vi "hioki.vi"(6 "TimeOut":u32=1000, 7 "PWA(V)":dbl, 8 "error in (no error)":errorcluster, 9 "Clu_SEQ":T1, 10 "EnumFunction":T2(ring), 11 "VISA resource name out":refnum<visa-resource-name>="COM2") -> (0 "error out":errorcluster, 2 "read buffer":string, 3 "Visa_HiokiMeterOut":refnum<visa-resource-name>)   [LabVIEW 2016]
uses:
  <vilib>/Instr/_visa.llb/VISA Open Access Mode.ctl
panel:
  out "x >= y?":bool
  out "sum":u32
  out "x-y":u32
  out "MeassuredValue":dbl format="%#_6e"
  out "ComparisonResult":i32
  out "Status":i32
  out "ch":i32
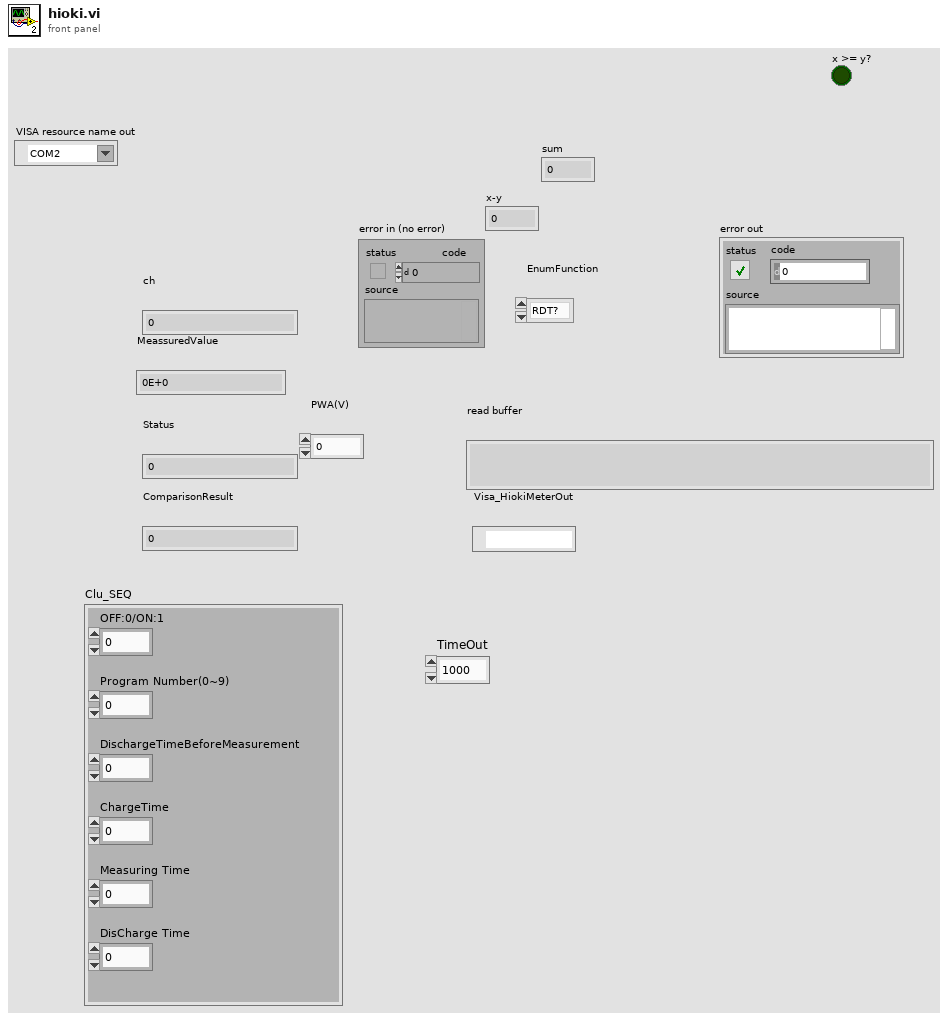
[diagram p1: front panel]
types:
  T1 = cluster{"OFF:0/ON:1":i32, "Program Number(0~9)":i32, "DischargeTimeBeforeMeasurement":dbl, "ChargeTime":dbl, "Measuring Time":dbl, "DisCharge Time":dbl}
  T2 = enum16{"RDT?", "IDN?", "SRT", "CBF", "SEQ?", "RMT", "SEQ", "PWS", "STP", "PWS?", "PWA", "CHS", ""}
  T3 = typedef "VISA Open Access Mode.ctl" = u32
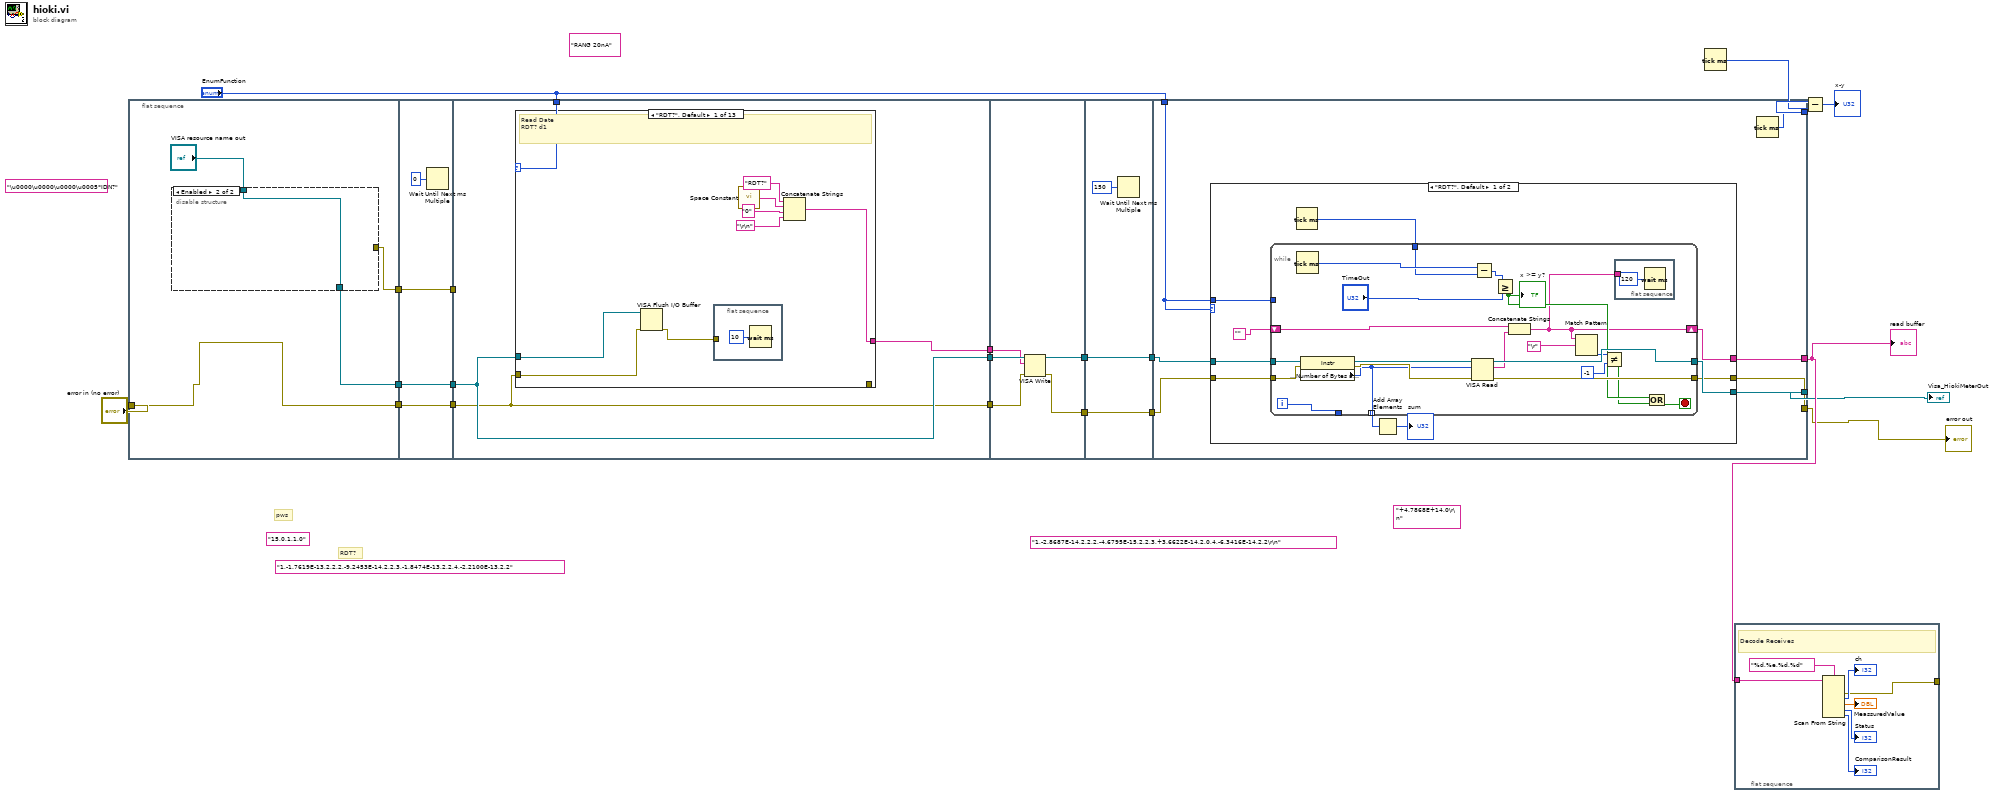
[diagram p0: block diagram]
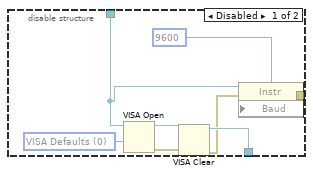
[diagram p2: hidden frame]
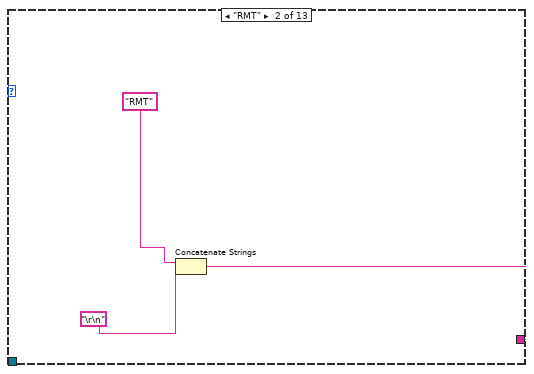
[diagram p3: hidden frame]
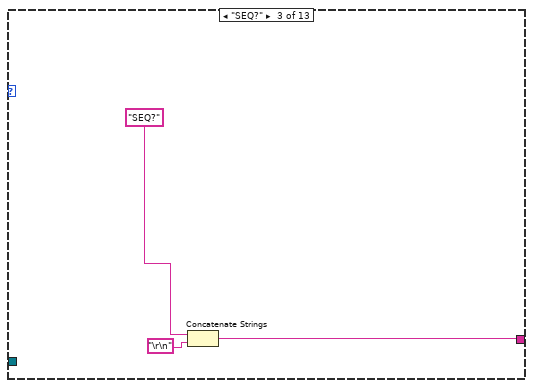
[diagram p4: hidden frame]
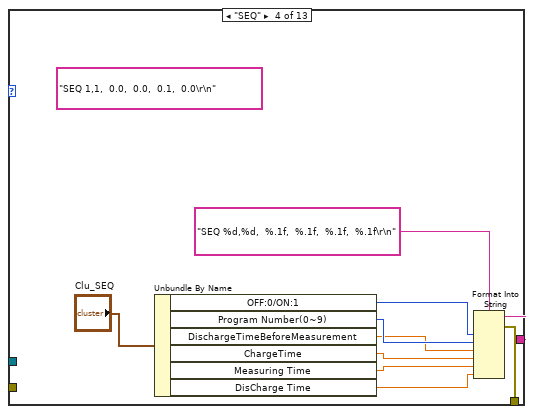
[diagram p5: hidden frame]
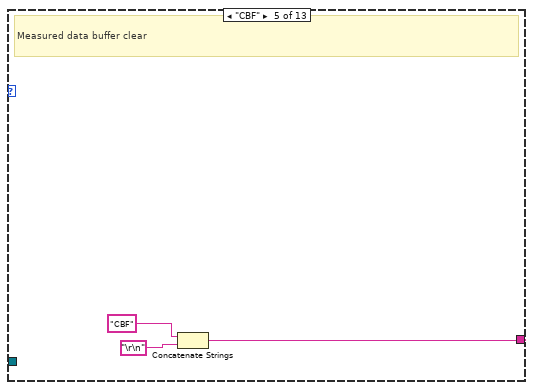
[diagram p6: hidden frame]
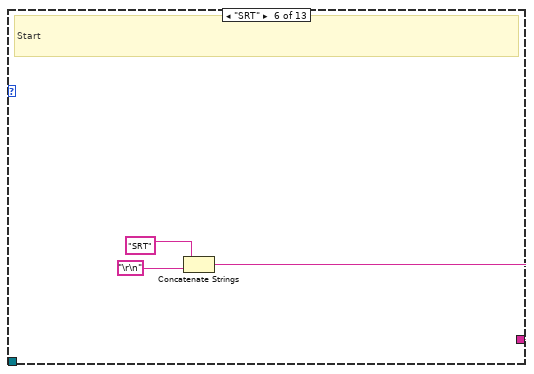
[diagram p7: hidden frame]
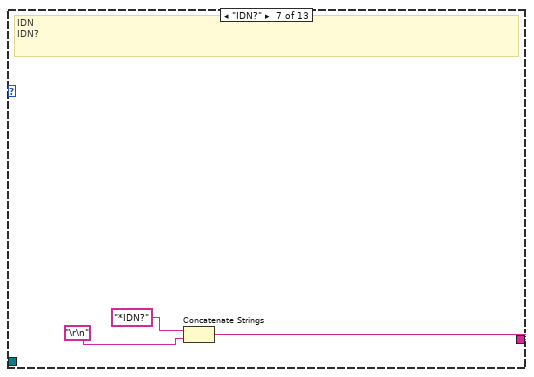
[diagram p8: hidden frame]
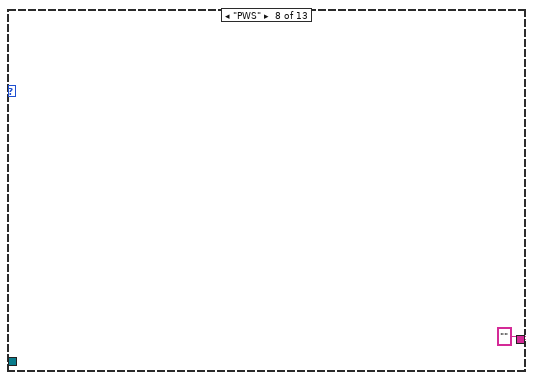
[diagram p9: hidden frame]
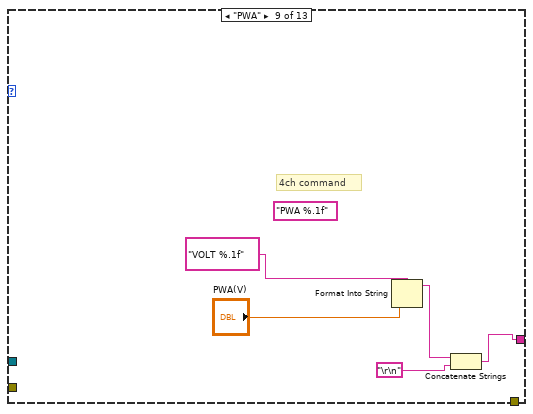
[diagram p10: hidden frame]
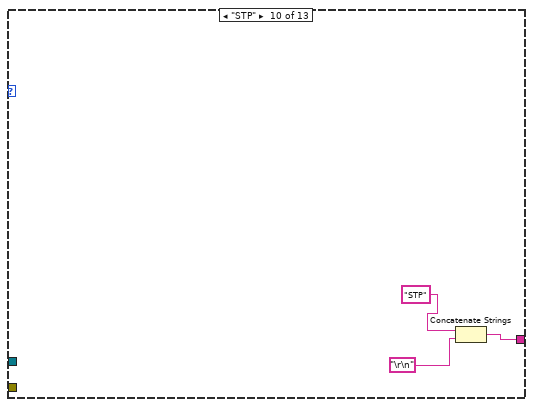
[diagram p11: hidden frame]
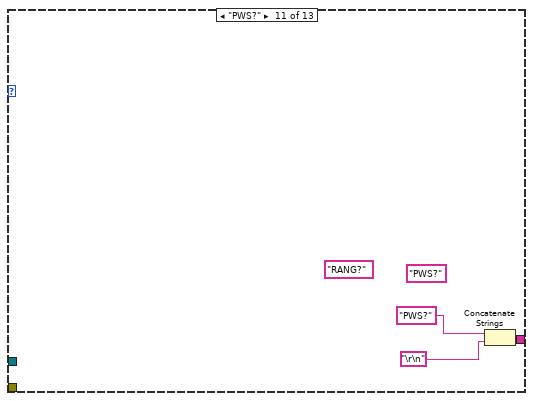
[diagram p12: hidden frame]
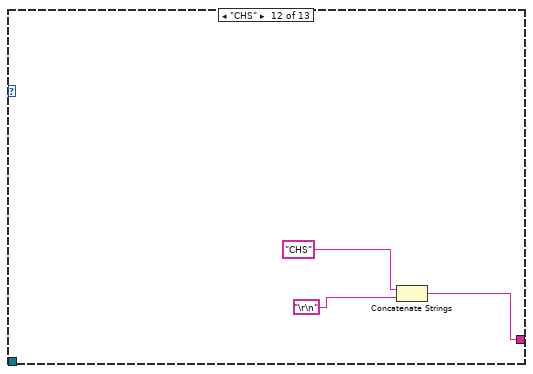
[diagram p13: hidden frame]
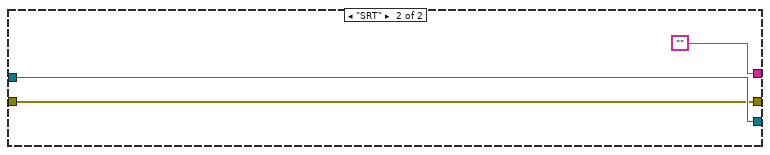
[diagram p15: hidden frame]
diagram:
  (unwired) "RANG 20nA"
  (unwired) "+4.7868E+14,0\r\n" ("read buffer 2")
  (unwired) "1,-2.8687E-14,2,2,2,-4.6795E-15,2,2,3,+3.6622E-14,2,0,4,-6.3416E-14,2,2\r\n" ("read buffer")
  (unwired) "1,-1.7619E-13,2,2,2,-9.2453E-14,2,2,3,-1.8474E-13,2,2,4,-2.2100E-13,2,2"
  (unwired) "15,0,1,1,0"
  (unwired) "\u0000\u0000\u0000\u0005*IDN?" ("Display")
  # "RDT?"
  # "pws"
  n1 = flat-sequence {
    tunnel: [w25] -> w8
    tunnel: [w24] -> w6
    tunnel: "error in (no error)" -> [w25]
    tunnel: [w22] -> w4
    tunnel: w8 -> [w38]
    tunnel: [w38] -> w7
    tunnel: w6 -> [w37]
    tunnel: [w37] -> w5
    tunnel: w4 -> [w36]
    tunnel: [w36] -> w3
    tunnel: w7 -> [w40]
    tunnel: w5 -> [w41]
    tunnel: "EnumFunction" -> [w42]
    tunnel: [w41] -> w18
    tunnel: [w40] -> w17
    tunnel: [w39] -> w14
    tunnel: w3 -> [_]
    tunnel: [w95] -> w19
    tunnel: w18 -> [w96]
    tunnel: w17 -> [w94]
    tunnel: [w93] -> w16
    tunnel: w14 -> [w92]
    tunnel: w19 -> [w99]
    tunnel: [w99] -> w21
    tunnel: w16 -> [w97]
    tunnel: [w97] -> w15
    tunnel: w21 -> [w106]
    tunnel: [w105] -> w2
    tunnel: [w104] -> w1
    tunnel: w15 -> [w103]
    tunnel: [w102] -> w9
    tunnel: "EnumFunction" -> [w101]
    tunnel: [w100] -> w12
    frame #0 {
      n2 = disable-structure shown="Enabled" {
        disable-tunnel: [w33 w34] -> w24
        disable-tunnel: "VISA resource name out" -> [w32 w34]
        disable-tunnel: [w31 _] -> w22
        frame Disabled {
          w28 = T3 0 items=["VISA Defaults"=0, "Exclusive Lock"=1, "Load Configured Settings"=4] ("Access Mode")
          n3 = VISA Open(access mode=w28, VISA resource name=w32) -> (VISA resource name=w30:refnum<visa-resource-name>, error out=w29:errorcluster)  [unwired: 3 in]
          n4 = VISA Clear(VISA resource name=w30, error in (no error)=w29) -> (VISA resource name out=w33:refnum<visa-resource-name>, error out=w26:errorcluster)
          n5 = property class="Instr"(reference=w32, error in=w26, "Baud"=u32 9600 ("Serial Settings:Baud Rate")) -> (error out=w31:errorcluster)  [unwired: 1 out]
        }
        frame Enabled {
        }
      }
    }
    frame #1 {
      n6 = Wait Until Next ms Multiple(millisecond multiple=u32 0) -> ()  [unwired: 1 out]
    }
    frame #2 {
      n7 = case shown="\"RDT?\", Default" w42 {
        tunnel: [w48 w53 w55 w66 w69 w72 w76 "" w79 w85 w86 w89 _] -> w39
        tunnel: [_ _ _ w65 _ _ _ _ _ _ _ _ _] -> _
        tunnel: w41 -> [w45 _ _ _ _ _ _ _ _ _ _ _ _]
        tunnel: w40 -> [w44 _ _ _ _ _ _ _ _ _ _ _ _]
        frame "RDT?", Default {
          # "Read Date\nRDT? d1"
          n8 = VISA Flush I/O Buffer(VISA resource name=w45, error in (no error)=w44) -> (error out=w43:errorcluster)  [unwired: 1 in, 1 out]
          n9 = flat-sequence {
            tunnel: w43 -> [_]
            frame #0 {
              n10 = Wait (ms)(milliseconds to wait=u32 10) -> ()  [unwired: 1 out]
            }
          }
          n11 = call <vilib>:"Space Constant.vi"() -> ("String"=w49:string)
          n12 = Concatenate Strings("RDT?", w49, "0" ("string"), "\r\n") -> (w48:string)
        }
        frame "RMT" {
          n13 = Concatenate Strings("RMT", "\r\n") -> (w53:string)
        }
        frame "SEQ?" {
          n14 = Concatenate Strings("SEQ?", "\r\n") -> (w55:string)
        }
        frame "SEQ" {
          (unwired) "SEQ 1,1,  0.0,  0.0,  0.1,  0.0\r\n" ("read buffer")
          n15 = Unbundle By Name("Clu_SEQ") -> ("OFF:0/ON:1"=w63:i32, "Program Number(0~9)"=w62:i32, "DischargeTimeBeforeMeasurement"=w61:dbl, "ChargeTime"=w60:dbl, "Measuring Time"=w59:dbl, "DisCharge Time"=w58:dbl)
          n16 = Format Into String(format string="SEQ %d,%d,  %.1f,  %.1f,  %.1f,  %.1f\r\n" ("read buffer"), w63, w62, w61, w60, w59, w58) -> (resulting string=w66:string, error out=w65:errorcluster)  [unwired: 2 in]
        }
        frame "CBF" {
          # "Measured data buffer clear"
          n17 = Concatenate Strings("CBF", "\r\n") -> (w69:string)
        }
        frame "SRT" {
          # "Start"
          n18 = Concatenate Strings("SRT", "\r\n") -> (w72:string)
        }
        frame "IDN?" {
          # "IDN \nIDN?"
          n19 = Concatenate Strings("*IDN?", "\r\n") -> (w76:string)
        }
        frame "PWS" {
        }
        frame "PWA" {
          (unwired) "PWA %.1f"
          # "4ch command"
          n20 = Format Into String(format string="VOLT %.1f", "PWA(V)") -> (resulting string=w81:string)  [unwired: 2 in, 1 out]
          n21 = Concatenate Strings(w81, "\r\n") -> (w79:string)
        }
        frame "STP" {
          n22 = Concatenate Strings("STP", "\r\n") -> (w85:string)
        }
        frame "PWS?" {
          (unwired) "RANG?"
          (unwired) "PWS?"
          n23 = Concatenate Strings("PWS?", "\r\n") -> (w86:string)
        }
        frame "CHS" {
          n24 = Concatenate Strings("CHS", "\r\n") -> (w89:string)
        }
        frame "" {
        }
      }
    }
    frame #3 {
      n25 = VISA Write(VISA resource name=w96, write buffer=w92, error in (no error)=w94) -> (VISA resource name out=w93:refnum<visa-resource-name>, error out=w95:errorcluster)  [unwired: 1 out]
    }
    frame #4 {
      n26 = Wait Until Next ms Multiple(millisecond multiple=u32 150) -> ()  [unwired: 1 out]
    }
    frame #5 {
      n27 = case shown="\"RDT?\", Default" w101 {
        tunnel: w106 -> [w116 w140]
        tunnel: [w115 w141] -> w105
        tunnel: [w114 w140] -> w104
        tunnel: w103 -> [w113 w141]
        tunnel: [w110 ""] -> w102
        tunnel: w101 -> [w109 _]
        frame "RDT?", Default {
          n28 = Tick Count (ms)() -> (millisecond timer value=w112:u32)
          n29 = while {
            tunnel: w112 -> [w130]
            tunnel: w116 -> [w137]
            tunnel: [w133] -> w114
            shift-right: [w118] -> w110
            shift-left: "" -> [w126]
            tunnel: w109 -> [_]
            tunnel: w113 -> [w132]
            tunnel: [w134] -> w115
            tunnel: [w119] -> _
            tunnel: [w117] -> w108 mode=indexing
            i -> [w119]
            stop <- w121 stop-if-true
            n30 = Tick Count (ms)() -> (millisecond timer value=w131:u32)
            n31 = property class="Instr"(reference=w132, error in=w137) -> (reference out=w136:refnum<visa-resource-name>, error out=w135:errorcluster, "Serial Settings:Number of Bytes at Serial Port"=w117:u32)
            n32 = VISA Read(VISA resource name=w136, byte count=w117, error in (no error)=w135) -> (VISA resource name out=w134:refnum<visa-resource-name>, read buffer=w127:string, error out=w133:errorcluster)  [unwired: 1 out]
            n33 = Subtract(x=w131, y=w130) -> (x-y=w129:u32)
            n34 = Greater Or Equal?(x=w129, y="TimeOut") -> (x >= y?=w125:bool)
            "x >= y?" <- w125
            n35 = Concatenate Strings(w126, w127) -> (w118:string)
            n36 = Match Pattern(string=w118, regular expression="\r") -> (offset past match=w124:i32)  [unwired: 1 in, 3 out]
            n37 = Not Equal?(x=w124, y=-1) -> (x != y?=w122:bool)
            n38 = flat-sequence {
              tunnel: w118 -> [_]
              frame #0 {
                n39 = Wait (ms)(milliseconds to wait=u32 120) -> ()  [unwired: 1 out]
              }
            }
            n40 = Or(x=w125, y=w122) -> (x .or. y?=w121:bool)
          }
          n41 = Add Array Elements(numeric array=w108) -> (sum=→"sum":u32)
        }
        frame "SRT" {
        }
      }
      n42 = Tick Count (ms)() -> (millisecond timer value=w100:u32)
    }
  }
  n43 = Tick Count (ms)() -> (millisecond timer value=w11:u32)
  n44 = flat-sequence {
    tunnel: w9 -> [w143]
    tunnel: [w142] -> _
    frame #0 {
      # "Decode Receives"
      n45 = Scan From String(format string="%d,%e,%d,%d", input string=w143) -> (error out=w142:errorcluster, output 1=→"ch":i32, output 2=→"MeassuredValue":dbl, output 3=→"Status":i32, output 4=→"ComparisonResult":i32)  [unwired: 6 in, 2 out]
    }
  }
  n46 = Subtract(x=w12, y=w11) -> (x-y=→"x-y":u32)
  "error out" <- w1
  "read buffer" <- w9
  "Visa_HiokiMeterOut" <- w2
